vi "ELVIS III v1.0 RPC Register Abort.vi"(8 "error in (no error)":errorcluster, 11 "Session":u32) -> (0 "error out":errorcluster)   [LabVIEW 2021]
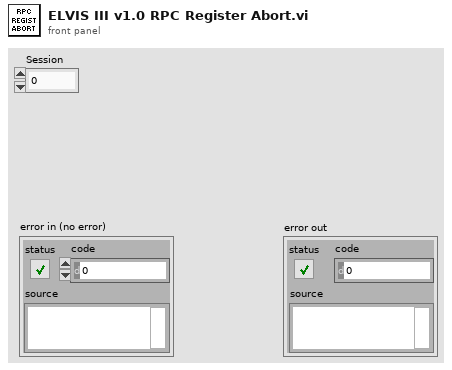
[diagram p1: front panel]
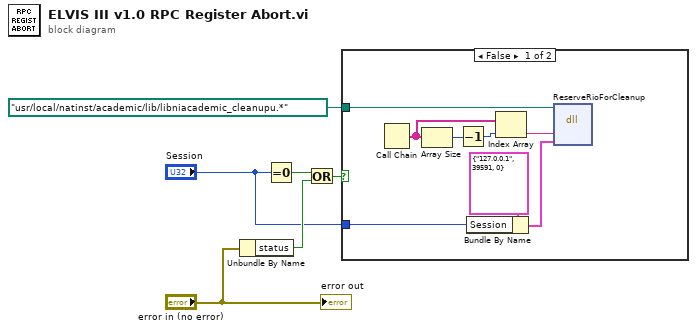
[diagram p0: block diagram]
diagram:
  n1 = Unbundle By Name("error in (no error)") -> ("status"=w6:bool)
  n2 = Equal To 0?(x="Session") -> (x = 0?=w5:bool)
  n3 = Or(x=w5, y=w6) -> (x .or. y?=w3:bool)
  n4 = case shown="False" w3 {
    tunnel: "Session" -> [w8 _]
    tunnel: path "/usr/local/natinst/academic/lib/libniacademic_cleanupu.*" ("path in") -> [w14 _]
    frame False {
      n5 = Call Chain() -> (call chain=w11:string[])
      n6 = Array Size(array=w11) -> (size(s)=w13:i32)
      n7 = Decrement(x=w13) -> (x-1=w12:i32)
      n8 = Bundle By Name(cluster=cluster{"IP":string, "Port":u16, "Session":u32} {"IP"="127.0.0.1", "Port"=39591, "Session"=0}, "Session"=w8) -> (w7:cluster{"IP":string, "Port":u16, "Session":u32})
      n9 = Index Array(array=w11, index=w12) -> (element=w10:string)
      n10 = dll-call lib="?" fn="ReserveRioForCleanup"(path in=w14, "topVIName"=w10, "resourcesInfo"=w7) -> ()  [unwired: 5 in, 2 out]
    }
    frame True {
      # "Session is invalid i.e. call from rpc server\nor error happens"
    }
  }
  "error out" <- "error in (no error)"
